vi "StopMusicLoop.vi"(8 "error in (no error)":errorcluster, 11 "Engine in":refnum<class "Engine.lvclass">) -> (0 "error out":errorcluster, 3 "Engine out":refnum<class "Engine.lvclass">)   [LabVIEW 2019, in "RT_Game.lvlib" / "Engine.lvclass"]
uses:
  Engine.lvclass
  MessageCluster.ctl
  Engine.lvclass/Engine.ctl
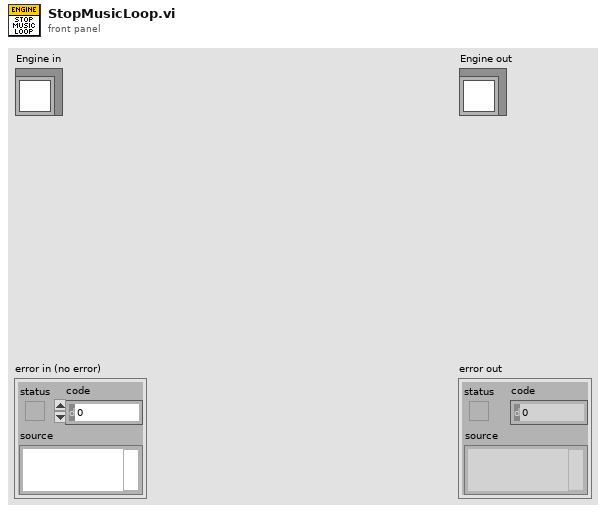
[diagram p1: front panel]
types:
  T1 = typedef "RT_Game.lvlib/Engine.lvclass/MessageCluster.ctl" = cluster{"Message":string, "Data":variant}
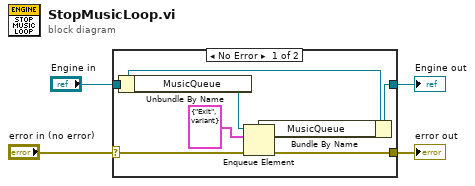
[diagram p0: block diagram]
diagram:
  n1 = case shown="No Error" "error in (no error)" {
    selector: "error in (no error)" -> [w8 w13]
    tunnel: [w7 w13] -> w3
    tunnel: [w6 w12] -> w1
    tunnel: "Engine in" -> [w5 w12]
    frame No Error {
      n2 = Unbundle By Name(w5) -> ("MusicQueue"=w9:refnum<queue>)
      n3 = Enqueue Element(queue=w9, element=T1 {"Message"="Exit", "Data"=variant}, error in (no error)=w8) -> (queue out=w10:refnum<queue>, error out=w7:errorcluster)  [unwired: 1 in, 1 out]
      n4 = Bundle By Name(cluster=w5, "MusicQueue"=w10) -> (w6:refnum<class "Engine.lvclass">)
    }
    frame Error {
    }
  }
  "error out" <- w3
  "Engine out" <- w1
